vi "Pre Launch Init.vi"(11 "PID Controller in":refnum<class "PID Controller.lvclass">) -> (0 "error out":errorcluster, 3 "PID Controller out":refnum<class "PID Controller.lvclass">)   [LabVIEW 2024, in "PID Controller.lvlib" / "PID Controller.lvclass"]
doc: "<p>(<strong>Filename</strong>: <span class=\"dnl\">Actor Framework.lvlib:Actor.lvclass:Pre Launch Init.vi</span>)</p>\n<p>Defines behavior that occurs after the <a href=\"nihelplauncher://docs/csh?context=lvcore_lvcomm_af_launch_nested_actor\">Launch Nested Actor</a> method is invoked but before the actor's Actor Core method begins running.</p>\n<p>By default, this method does nothing. A descendant class may override it to define behavior.</p>"
uses:
  PID Controller.lvclass
  PID Controller.lvclass/PID Controller.ctl
  <vilib>/ActorFramework/Actor/Actor.lvclass
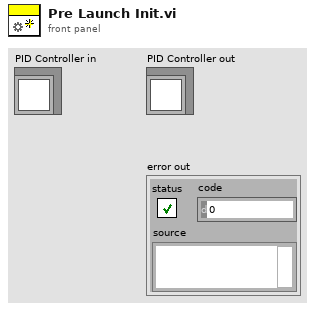
[diagram p1: front panel]
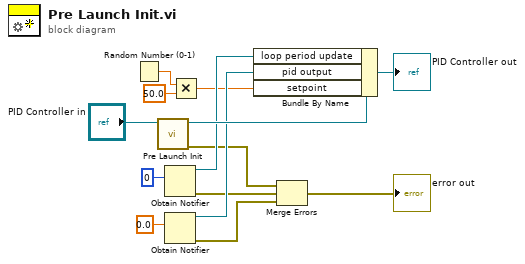
[diagram p0: block diagram]
diagram:
  n1 = Random Number (0-1)() -> (number: 0 to 1=w9:dbl)
  n2 = call-parent "Pre Launch Init.vi"("Actor in"="PID Controller in") -> ("error out"=w4:errorcluster, "Actor out"=w12:refnum<class "PID Controller.lvclass">)  [unwired: 9 in]
  n3 = Obtain Notifier(notification data type=u32 0) -> (notifier out=w7:refnum<notifier>, error out=w6:errorcluster)  [unwired: 3 in, 1 out]
  n4 = Obtain Notifier(notification data type=0.0) -> (notifier out=w11:refnum<notifier>, error out=w5:errorcluster)  [unwired: 3 in, 1 out]
  n5 = Multiply(x=w9, y=50.0) -> (x*y=w2:dbl)
  n6 = Bundle By Name(cluster=w12, "loop period update"=w7, "pid output"=w11, "setpoint"=w2) -> (→"PID Controller out":refnum<class "PID Controller.lvclass">)
  n7 = Merge Errors(w4, w6, w5) -> (→"error out":errorcluster)
